vi "RGB to GRB rev.vi"(9 "ID":u8, 11 "Element":u32) -> (1 "Valid":bool, 2 "Array":bool[](array[boolean]), 3 "Reset":bool)   [LabVIEW 2015]
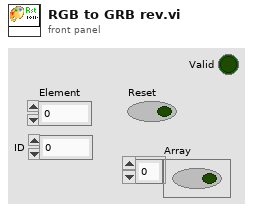
[diagram p1: front panel]
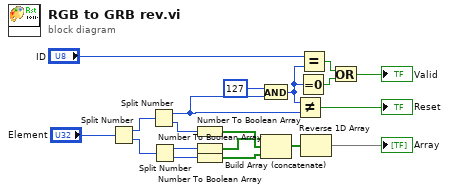
[diagram p0: block diagram]
diagram:
  n1 = Split Number(x="Element") -> (hi(x)=w10:u16, lo(x)=w11:u16)
  n2 = Split Number(x=w10) -> (hi(x)=w7:u8, lo(x)=w12:u8)
  n3 = Split Number(x=w11) -> (hi(x)=w13:u8, lo(x)=w14:u8)
  n4 = Number To Boolean Array(number=w12) -> (Boolean array=w16:bool[])
  n5 = Number To Boolean Array(number=w13) -> (Boolean array=w15:bool[])
  n6 = Number To Boolean Array(number=w14) -> (Boolean array=w17:bool[])
  n7 = And(x=u8 127, y=w7) -> (x .and. y?=w1:u8)
  n8 = Build Array (concatenate)(w15, w16, w17) -> (w18:bool[])
  n9 = Not Equal?(x=w1, y=w7) -> (x != y?=→"Reset":bool)
  n10 = Equal To 0?(x=w1) -> (x = 0?=w2:bool)
  n11 = Equal?(x="ID", y=w1) -> (x = y?=w5:bool)
  n12 = Reverse 1D Array(array=w18) -> (reversed array=→"Array":bool[])
  n13 = Or(x=w5, y=w2) -> (x .or. y?=→"Valid":bool)
